vi "Close SHVs.vi"(8 "error in (no error)":errorcluster, 11 "Freezer in":refnum<class "Freezer.lvclass">) -> (0 "error out":errorcluster, 3 "Freezer out":refnum<class "Freezer.lvclass">)   [LabVIEW 2015, in "cRIO-Carbondioxide.lvlib" / "CO2-Actor.lvlib" / "Freezer.lvclass"]
uses:
  Freezer.lvclass
  Freezer.lvclass/Freezer.ctl
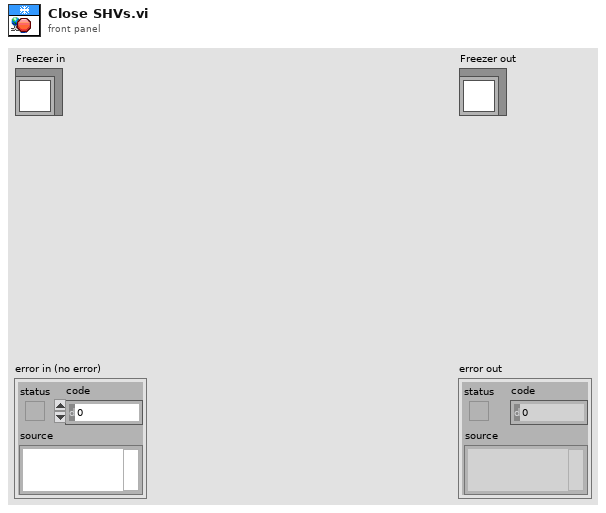
[diagram p1: front panel]
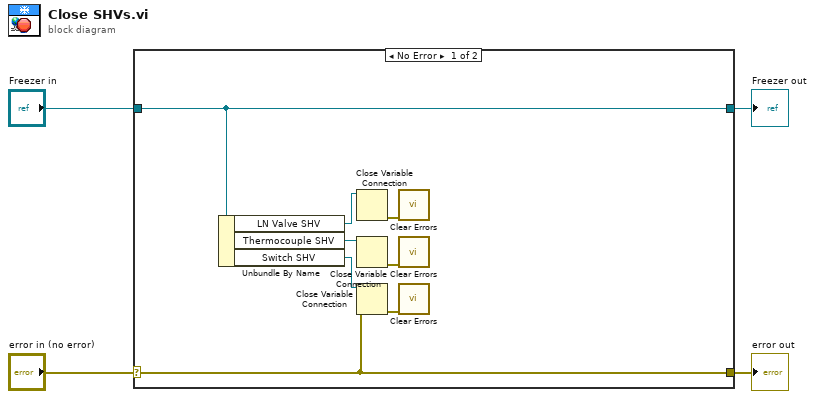
[diagram p0: block diagram]
diagram:
  n1 = case shown="No Error" "error in (no error)" {
    selector: "error in (no error)" -> [w5 w14]
    tunnel: [w5 w14] -> w3
    tunnel: [w6 w13] -> w1
    tunnel: "Freezer in" -> [w6 w13]
    frame No Error {
      n2 = Unbundle By Name(w6) -> ("LN Valve SHV"=w9:refnum<k21>, "Thermocouple SHV"=w11:refnum<k21>, "Switch SHV"=w7:refnum<k21>)
      n3 = Close Variable Connection(11:w9) -> (0:w8:errorcluster)  [unwired: 1 in]
      n4 = Close Variable Connection(11:w11) -> (0:w10:errorcluster)  [unwired: 1 in]
      n5 = Close Variable Connection(8:w5, 11:w7) -> (0:w12:errorcluster)
      n6 = call <vilib>:"Clear Errors.vi"("error in (no error)"=w8) -> ()  [unwired: 5 in, 2 out]
      n7 = call <vilib>:"Clear Errors.vi"("error in (no error)"=w10) -> ()  [unwired: 5 in, 2 out]
      n8 = call <vilib>:"Clear Errors.vi"("error in (no error)"=w12) -> ()  [unwired: 5 in, 2 out]
    }
    frame Error {
    }
  }
  "error out" <- w3
  "Freezer out" <- w1
